vi "Lock Cluster Controls.vi"(8 "error in (no error)":errorcluster, 10 "Ctl Refnum in":refnum<vi>) -> (0 "error out":errorcluster, 2 "Ctl Refnum":refnum<vi>)   [LabVIEW 2020, in "VolatusGUIEditor.lvlib" / "Editor.lvclass"]
uses:
  Editor.lvclass
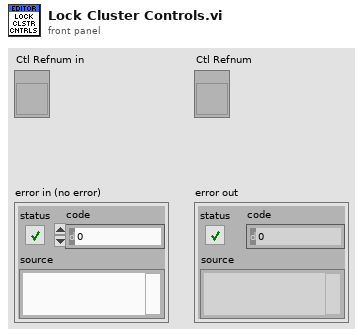
[diagram p1: front panel]
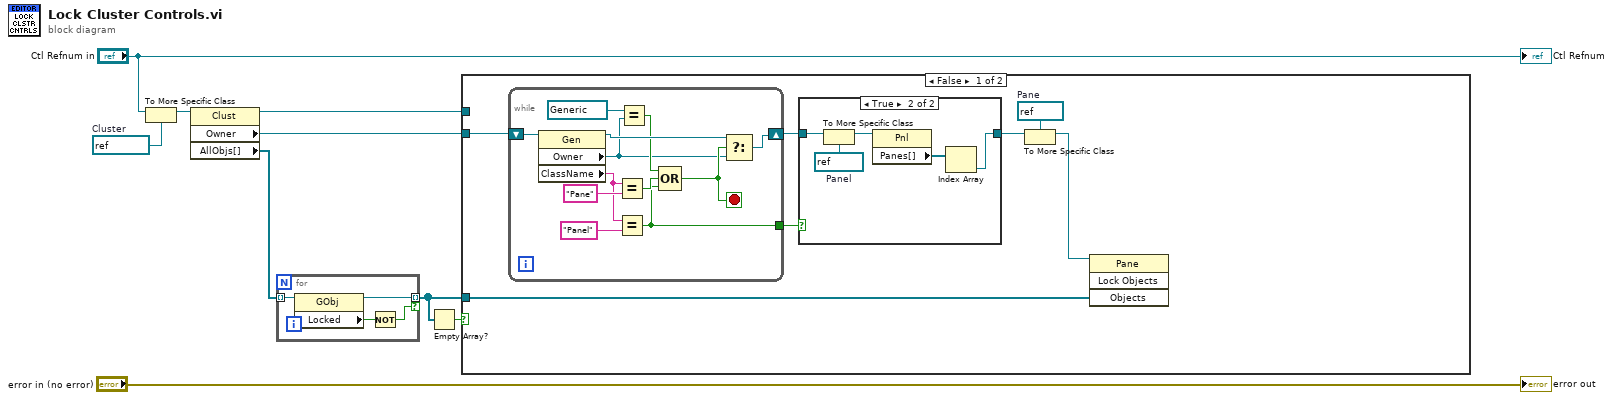
[diagram p0: block diagram]
diagram:
  w8 = refnum<vi> refnum  # Cluster
  n1 = To More Specific Class(target class=w8, reference="Ctl Refnum in") -> (specific class reference=w7:refnum<vi>)  [unwired: 1 in, 1 out]
  n2 = property class="Clust"(reference=w7) -> (reference out=w1:refnum<vi>, "Owner"=w2:refnum<vi>, "AllObjs[]"=w5:refnum<vi>[])  [unwired: 1 in, 1 out]
  n3 = for {
    tunnel: w5 -> [w13] mode=indexing
    tunnel: [w12] -> w4 mode=indexing if=w10
    n4 = property class="GObj"(reference=w13) -> (reference out=w12:refnum<vi>, "Locked"=w11:bool)  [unwired: 1 in, 1 out]
    n5 = Not(x=w11) -> (.not. x?=w10:bool)
  }
  n6 = Empty Array?(array=w4) -> (empty?=w3:bool)
  n7 = case shown="False" w3 {
    tunnel: w4 -> [w20 _]
    tunnel: w2 -> [w19 _]
    tunnel: w1 -> [_ _]
    frame False {
      w18 = refnum<vi> refnum  # Pane
      n8 = while {
        shift-right: [w35] -> w15
        shift-left: w19 -> [w38]
        tunnel: [w27] -> w16
        stop <- w32 stop-if-true
        n9 = property class="Gen"(reference=w38) -> (reference out=w36:refnum<vi>, "Owner"=w30:refnum<vi>, "ClassName"=w28:string)  [unwired: 1 in, 1 out]
        n10 = Equal?(x=w28, y="Pane") -> (x = y?=w33:bool)
        n11 = Equal?(x=w28, y="Panel") -> (x = y?=w27:bool)
        n12 = Equal?(x=refnum<vi> refnum, y=w30) -> (x = y?=w31:bool)
        n13 = Compound Arithmetic op=OR(w31, w33, w27) -> (w32:bool)
        n14 = Select(t=w36, s=w32, f=w30) -> (s? t:f=w35:refnum<vi>)
      }
      n15 = case shown="True" w16 {
        tunnel: w15 -> [w21 w26]
        tunnel: [w21 w22] -> w14
        frame False {
        }
        frame True {
          w25 = refnum<vi> refnum  # Panel
          n16 = To More Specific Class(target class=w25, reference=w26) -> (specific class reference=w24:refnum<vi>)  [unwired: 1 in, 1 out]
          n17 = property class="Pnl"(reference=w24) -> ("Panes[]"=w23:refnum<vi>[])  [unwired: 1 in, 2 out]
          n18 = Index Array(array=w23) -> (element=w22:refnum<vi>)  [unwired: 1 in]
        }
      }
      n19 = To More Specific Class(target class=w18, reference=w14) -> (specific class reference=w17:refnum<vi>)  [unwired: 1 in, 1 out]
      n20 = invoke class="Pane" method="Lock Objects"(reference=w17, "Objects"=w20) -> ()  [unwired: 2 in, 4 out]
    }
    frame True {
    }
  }
  "error out" <- "error in (no error)"
  "Ctl Refnum" <- "Ctl Refnum in"
